vi "microFPGA_TTL_addr_24_ctrl.vi"(0 "VISA resource name":refnum<visa-resource-name>, 1 "TTL_channel":u16(ring)=3 items=["channel No 0", "channel No 1", "channel No 2", "channel No 3"], 2 "write or read":u16(ring) items=["read", "write"], 5 "TTL_mode_WRITE":u16(ring) items=["LO", "HIGH"], 11 "error in (no error)":errorcluster) -> (4 "VISA out":refnum<visa-resource-name>, 6 "TTL_mode_READ":u16(ring) items=["LO", "HIGH"], 8 "value confirm":bool=TRUE, 10 "abort_wrong_input":bool, 15 "error out":errorcluster)   [LabVIEW 2021]
panel:
  out "mode read string answer":string
  out "mode read string":string
  out "mode write string":string
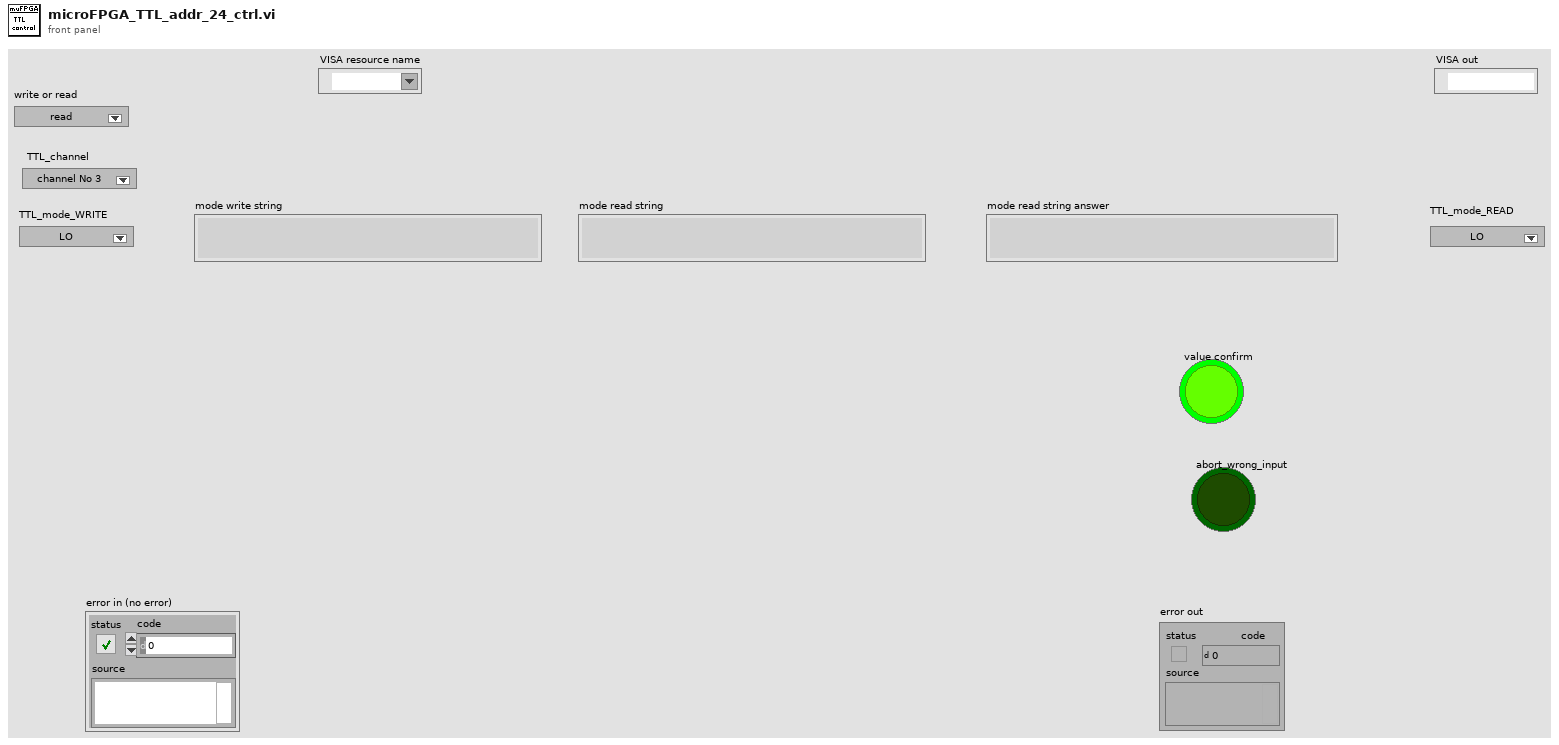
[diagram p1: front panel]
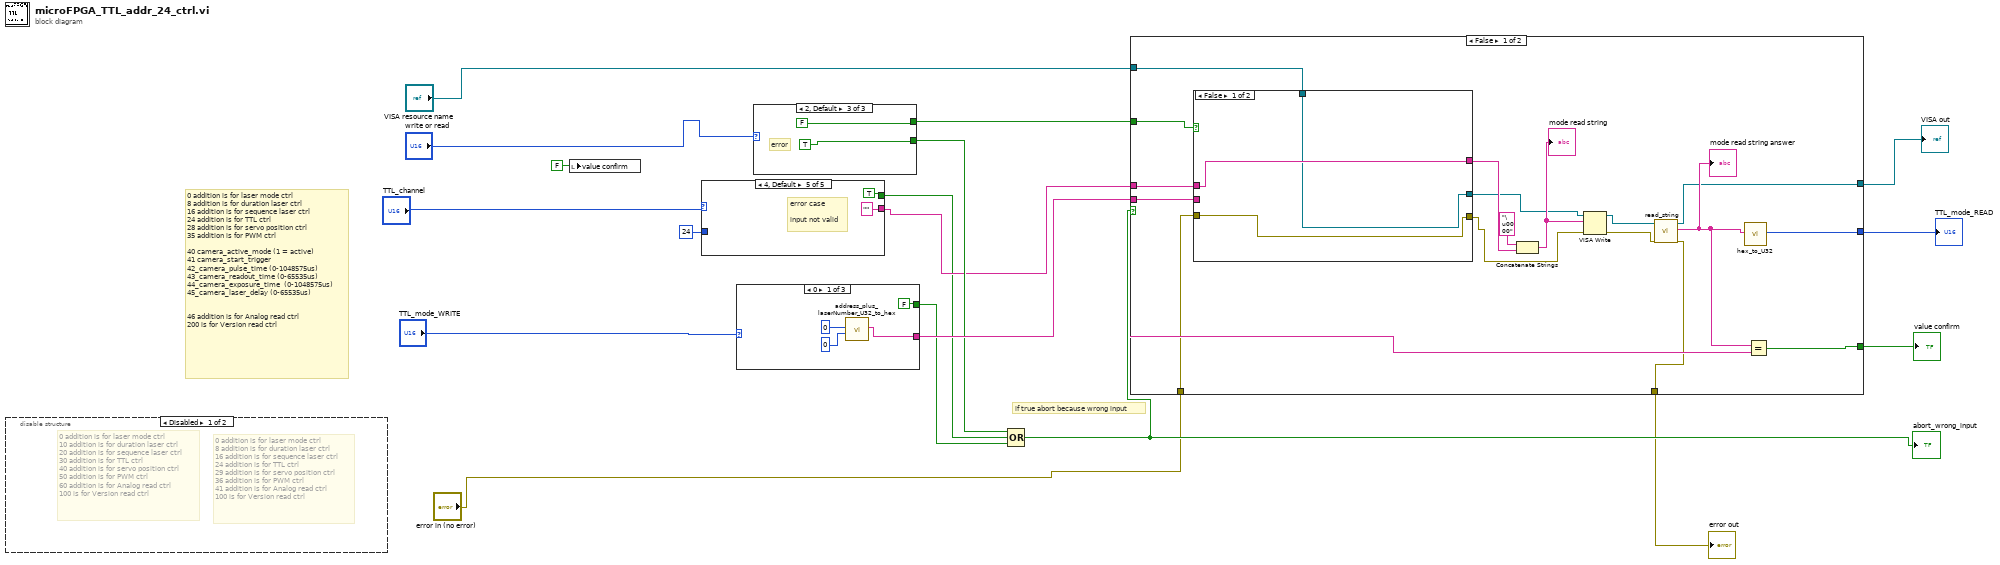
[diagram p0: block diagram]
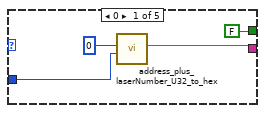
[diagram p3: hidden frame]
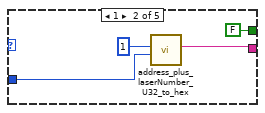
[diagram p4: hidden frame]
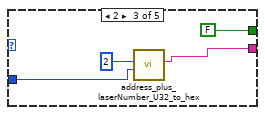
[diagram p5: hidden frame]
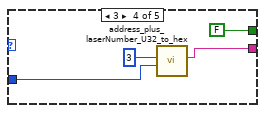
[diagram p6: hidden frame]
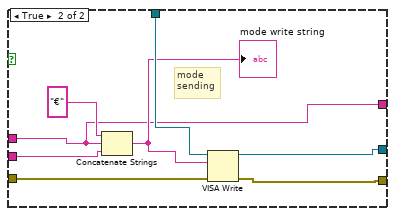
[diagram p7: hidden frame]
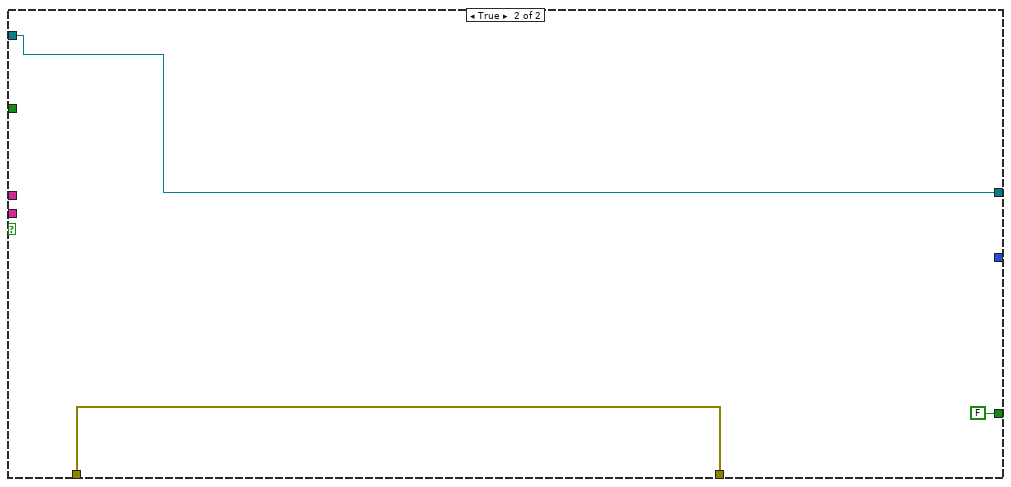
[diagram p8: hidden frame]
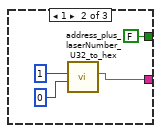
[diagram p9: hidden frame]
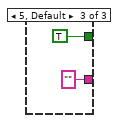
[diagram p10: hidden frame]
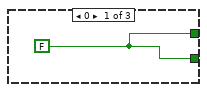
[diagram p11: hidden frame]
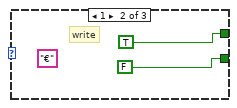
[diagram p12: hidden frame]
diagram:
  # "0 addition is for laser mode ctrl\n8 addition is for duration laser ctrl\n16 addition is for sequence laser ctrl\n24 addition is for TTL ctrl\n28 addition is for servo position ctrl\n35 addition is for PWM ctrl\n\n40 camera_active_mode (1 = active) \n41 camera_start_trigger\n42_camera_pulse_time (0-1048575us)\n43_camera_readout_time (0-65535us)\n44_camera_exposure_time  (0-1048575us)\n45_camera_laser_delay (0-65535us)\n\n\n46 addition is for Analog read ctrl\n200 is for Version read ctrl"
  # "if true abort because wrong input"
  n1 = disable-structure shown="Disabled" {
    frame Disabled {
      # "0 addition is for laser mode ctrl\n8 addition is for duration laser ctrl\n16 addition is for sequence laser ctrl\n24 addition is for TTL ctrl\n29 addition is for servo position ctrl\n36 addition is for PWM ctrl\n41 addition is for Analog read ctrl\n100 is for Version read ctrl"
      # "0 addition is for laser mode ctrl\n10 addition is for duration laser ctrl\n20 addition is for sequence laser ctrl\n30 addition is for TTL ctrl\n40 addition is for servo position ctrl\n50 addition is for PWM ctrl\n60 addition is for Analog read ctrl\n100 is for Version read ctrl"
    }
    frame Enabled {
    }
  }
  n2 = local write "value confirm"(FALSE ("value confirm")) -> ()
  n3 = case shown="4, Default" "TTL_channel" {
    tunnel: [w20 w24 w28 w32 "" ("string 5")] -> w3
    tunnel: [FALSE FALSE FALSE FALSE TRUE] -> w2
    tunnel: u32 24 ("adress offset") -> [w19 w23 w27 w31 _]
    frame 0 {
      n4 = call "address_plus_laserNumber_U32_to_hex.vi"("adress offset"=w19, "y 3"=u32 0) -> ("string 5"=w20:string)  [unwired: 8 in]
    }
    frame 1 {
      n5 = call "address_plus_laserNumber_U32_to_hex.vi"("adress offset"=w23, "y 3"=u32 1) -> ("string 5"=w24:string)  [unwired: 8 in]
    }
    frame 2 {
      n6 = call "address_plus_laserNumber_U32_to_hex.vi"("adress offset"=w27, "y 3"=u32 2) -> ("string 5"=w28:string)  [unwired: 8 in]
    }
    frame 3 {
      n7 = call "address_plus_laserNumber_U32_to_hex.vi"("adress offset"=w31, "y 3"=u32 3) -> ("string 5"=w32:string)  [unwired: 8 in]
    }
    frame 4, Default {
      # "error case\n\ninput not valid"
    }
  }
  n8 = case shown="0" "TTL_mode_WRITE" {
    tunnel: [w37 w42 "" ("string 5")] -> w14
    tunnel: [FALSE FALSE TRUE] -> w10
    frame 0 {
      n9 = call "address_plus_laserNumber_U32_to_hex.vi"("adress offset"=u32 0, "y 3"=u32 0) -> ("string 5"=w37:string)  [unwired: 8 in]
    }
    frame 1 {
      n10 = call "address_plus_laserNumber_U32_to_hex.vi"("adress offset"=u32 0, "y 3"=u32 1) -> ("string 5"=w42:string)  [unwired: 8 in]
    }
    frame 5, Default {
    }
  }
  n11 = case shown="2, Default" "write or read" {
    tunnel: [w47 TRUE FALSE] -> w15
    tunnel: [w47 FALSE TRUE] -> w11
    frame 0 {
      w47 = FALSE
    }
    frame 1 {
      (unwired) "€" ("hex")
      # "write"
    }
    frame 2, Default {
      # "error"
    }
  }
  n12 = Compound Arithmetic op=OR(w11, w2, w10) -> (w8:bool)
  "abort_wrong_input" <- w8
  n13 = case shown="False" w8 {
    tunnel: "VISA resource name" -> [w68 w81]
    tunnel: w3 -> [w65 _]
    tunnel: w15 -> [w59 _]
    tunnel: [w58 _] -> w5
    tunnel: w14 -> [w56 _]
    tunnel: [w55 FALSE] -> w13
    tunnel: [w54 w81] -> w9
    tunnel: "error in (no error)" -> [w53 w80]
    tunnel: [w52 w80] -> w6
    frame False {
      n14 = case shown="False" w59 {
        tunnel: w65 -> [w71 w76]
        tunnel: w68 -> [w70 w78]
        tunnel: [w71 w76] -> w66
        tunnel: w56 -> [_ w75]
        tunnel: [w70 w74] -> w61
        tunnel: [w69 w73] -> w60
        tunnel: w53 -> [w69 w72]
        frame False {
        }
        frame True {
          # "mode \nsending"
          n15 = Concatenate Strings("€" ("string"), w76, w75) -> (w77:string)
          "mode write string" <- w77
          n16 = VISA Write(VISA resource name=w78, write buffer=w77, error in (no error)=w72) -> (VISA resource name out=w74:refnum<visa-resource-name>, error out=w73:errorcluster)  [unwired: 1 out]
        }
      }
      n17 = Concatenate Strings("\u0000" ("string"), w66) -> (w64:string)
      "mode read string" <- w64
      n18 = VISA Write(VISA resource name=w61, write buffer=w64, error in (no error)=w60) -> (VISA resource name out=w63:refnum<visa-resource-name>, error out=w62:errorcluster)  [unwired: 1 out]
      n19 = call "read_string.vi"("error in (no error)"=w62, "VISA resource name 2"=w63) -> ("error out"=w52:errorcluster, "read buffer"=w57:string, "VISA resource name"=w54:refnum<visa-resource-name>)  [unwired: 7 in]
      "mode read string answer" <- w57
      n20 = call "hex_to_U32.vi"("hex"=w57) -> ("U32"=w58:u32)  [unwired: 9 in]
      n21 = Equal?(x=w57, y=w56) -> (x = y?=w55:bool)
    }
    frame True {
    }
  }
  "value confirm" <- w13
  "VISA out" <- w9
  "error out" <- w6
  "TTL_mode_READ" <- w5
